vi "Get Application Instance Name.vi"(11 "VI Type":refnum<class "Standard VI Type.lvclass">) -> (3 "Name":string)   [LabVIEW 2020, in "Peek Window.lvlib"]
uses:
  Peek Window.lvlib
  VI Types/Standard VI Type/Standard VI Type.lvclass
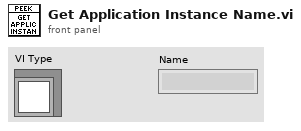
[diagram p1: front panel]
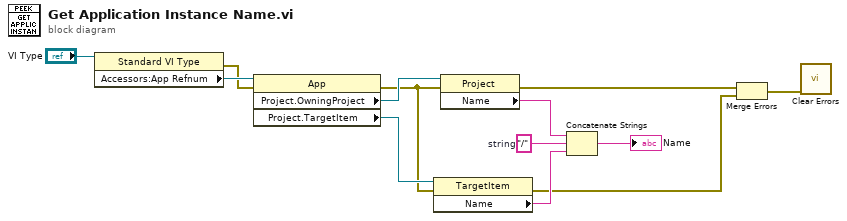
[diagram p0: block diagram]
diagram:
  w9 = "/"  # string
  n1 = property class="Standard VI Type"(reference="VI Type") -> (error out=w1:errorcluster, "Accessors:App Refnum"=w2:refnum<vi>)  [unwired: 1 in, 1 out]
  n2 = property class="App"(reference=w2, error in=w1) -> (error out=w7:errorcluster, "Project.OwningProject"=w13:refnum<vi>, "Project.TargetItem"=w12:refnum<vi>)  [unwired: 1 out]
  n3 = property class="TargetItem"(reference=w12, error in=w7) -> (error out=w5:errorcluster, "Name"=w10:string)  [unwired: 1 out]
  n4 = property class="Project"(reference=w13, error in=w7) -> (error out=w6:errorcluster, "Name"=w11:string)  [unwired: 1 out]
  n5 = Concatenate Strings(w11, w9, w10) -> (→"Name":string)
  n6 = Merge Errors(w6, w5) -> (w4:errorcluster)
  n7 = call <vilib>:"Clear Errors.vi"("error in (no error)"=w4) -> ()  [unwired: 5 in, 2 out]
